vi "Real Matrix Trace.vi"(0 "Input Matrix":T1) -> (1 "trace":dbl format="%.2f", 2 "error":i32)   [LabVIEW 2024, in "NI_AALPro.lvlib"]
doc: "<p>Finds the <strong>trace</strong> of <strong>Input Matrix</strong>. Wire data to the <strong>Input Matrix</strong> input to determine the polymorphic instance to use or <a href=\"nihelplauncher://docs/csh?context=lvcore_lvhowto_selectingdefaultinstpolyvi\">manually select</a> the instance.</p>"
uses:
  NI_AALPro.lvlib
  RealMatrix.ctl
  <resource>/lvanlys.dll
  NI_Matrix.lvlib
panel:
  # "Trace"
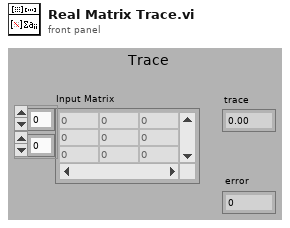
[diagram p1: front panel]
types:
  T1 = typedef "NI_Matrix.lvlib/RealMatrix.ctl" = dbl[][]
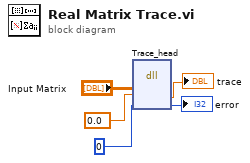
[diagram p0: block diagram]
diagram:
  n1 = dll-call lib="C:/Program Files (x86)/National Instruments/LabVIEW 2024/resource/lvanlys.*" fn="Trace_head"("Input Matrix"="Input Matrix", 0.0, 0) -> (→"trace":dbl, →"error":i32)  [unwired: 5 in, 2 out]
